vi "Calib_read_files.vi"   [LabVIEW 2013]
uses:
  Globals/Calib_global.vi
types:
  T1 = typedef "Cal_Inst_type.ctl" = enum16{"Propeller anemometer", "Pressure Transducer", "Hot wire", "Cross wire velocity", "Cross wire angle", "Generic Linear", "Generic Polynomial", "Generic BackPoly", "Fast FID", "Thermocouple", "Cold wire", "Pulsed Wire"}
  T2 = typedef "TypeCalib.ctl" = cluster{"high limit (10V)":sgl, "low limit (-10V)":sgl, "Ch No":i16, "Var name":string, "DAQmx Chan":tag}
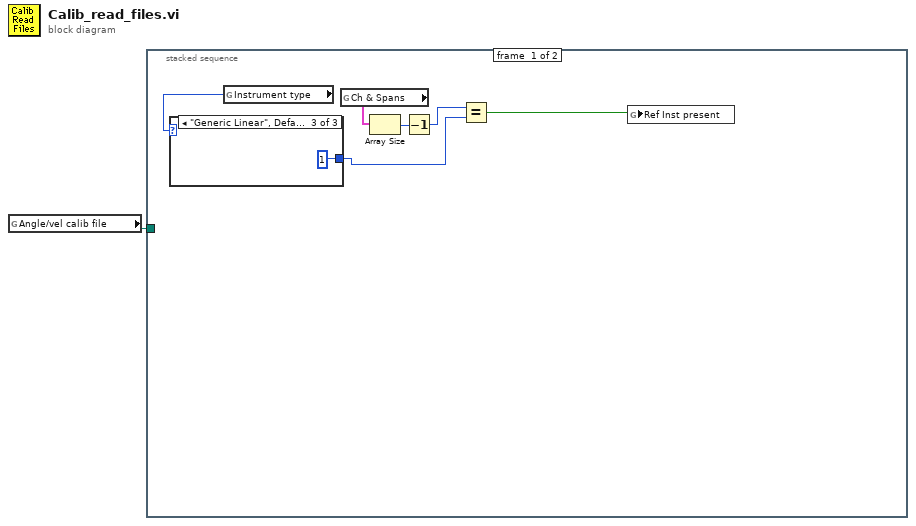
[diagram p0: block diagram]
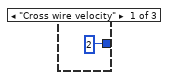
[diagram p2: hidden frame]
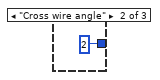
[diagram p3: hidden frame]
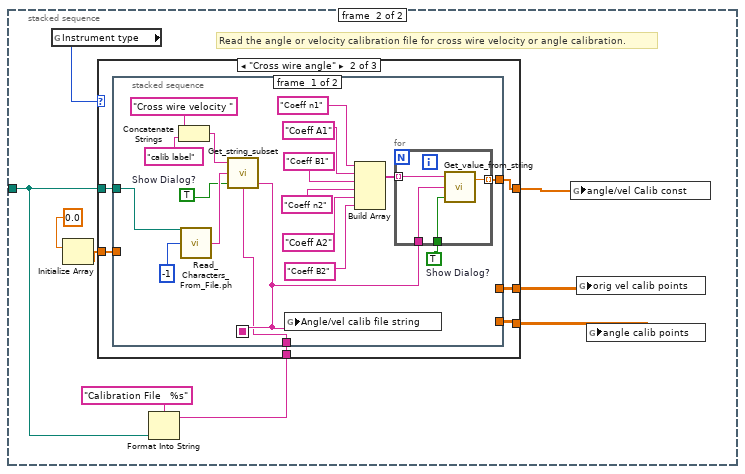
[diagram p4: hidden frame]
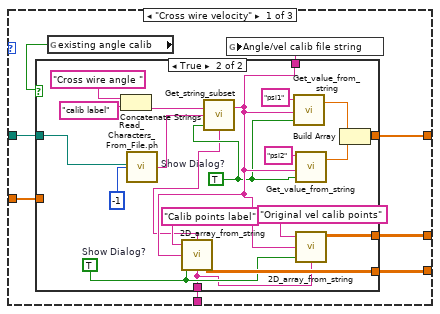
[diagram p5: hidden frame]
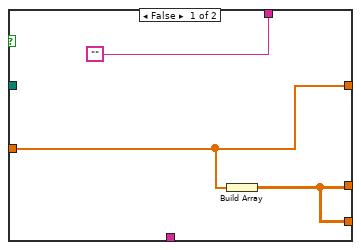
[diagram p6: hidden frame]
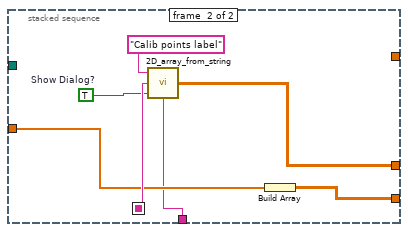
[diagram p7: hidden frame]
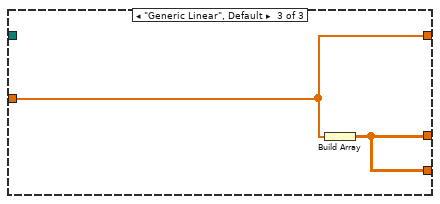
[diagram p8: hidden frame]
diagram:
  n1 = global read "Calib_global.vi" "Angle/vel calib file"() -> (w1:path)
  n2 = stacked-sequence {
    tunnel: w1 -> [_ w12]
    frame #0 {
      n3 = global read "Calib_global.vi" "Instrument type"() -> (w7:T1)
      n4 = case shown="\"Generic Linear\", Default" w7 {
        tunnel: [2 2 1] -> w2
        frame "Cross wire velocity" {
        }
        frame "Cross wire angle" {
        }
        frame "Generic Linear", Default {
        }
      }
      n5 = global read "Calib_global.vi" "Ch & Spans"() -> (w5:T2[])
      n6 = Array Size(array=w5) -> (size(s)=w6:i32)
      n7 = Decrement(x=w6) -> (x-1=w4:i32)
      n8 = Equal?(x=w4, y=w2) -> (x = y?=w3:bool)
      n9 = global write "Calib_global.vi" "Ref Inst present"(w3) -> ()
    }
    frame #1 {
      # "Read the angle or velocity calibration file for cross wire velocity or angle calibration."
      n10 = global read "Calib_global.vi" "Instrument type"() -> (w17:T1)
      n11 = Initialize Array(0.0) -> (w19:dbl[])  [unwired: 1 out]
      n12 = Format Into String(format string="Calibration File   %s", w12) -> (resulting string=w11:string)  [unwired: 2 in, 1 out]
      n13 = case shown="\"Cross wire angle\"" w17 {
        tunnel: [w27 w51 w86] -> w18
        tunnel: w19 -> [w26 w54 w86]
        tunnel: [w24 w55 w85] -> w14
        tunnel: [w25 w53 w85] -> w15
        tunnel: w12 -> [w21 w52 _]
        tunnel: w11 -> [w20 w50 _]
        frame "Cross wire velocity" {
          n14 = global read "Calib_global.vi" "existing angle calib"() -> (w23:bool)
          n15 = case shown="True" w23 {
            tunnel: [w30 w40] -> w27
            tunnel: w26 -> [w30 _]
            tunnel: [w29 w38] -> w25
            tunnel: [w29 w36] -> w24
            tunnel: ["" w35] -> w22
            tunnel: w21 -> [_ w34]
            tunnel: w20 -> [_ w31]
            frame False {
              n16 = Build Array(w30) -> (w29:dbl[][])
            }
            frame True {
              w32 = TRUE  # Show Dialog?
              w33 = TRUE  # Show Dialog?
              n17 = Concatenate Strings("Cross wire angle ", "calib label") -> (w41:string)
              n18 = call "Read_Characters_From_File.ph.vi"("file path (dialog if empty)"=w34, "number of characters (all:-1)"=-1) -> ("character string"=w43:string)  [unwired: 7 out]
              n19 = call "Get_string_subset.vi"("String Name"=w31, "Show Dialog?"=w33, "String to split"=w43, "File Label"=w41) -> ("Output string"=w35:string)  [unwired: 1 out]
              n20 = call "2D_array_from_string.vi"("String Name"=w31, "Show Dialog?"=w32, "Input string"=w35, "Array title"="Calib points label") -> ("2D data array"=w38:dbl[][])
              n21 = call "Get_value_from_string.vi"("Show Dialog?"=w33, "Input string"=w35, "Variable name"="psi1") -> ("Value"=w45:dbl)  [unwired: 1 out]
              n22 = call "Get_value_from_string.vi"("Show Dialog?"=w33, "Input string"=w35, "Variable name"="psi2") -> ("Value"=w44:dbl)  [unwired: 1 out]
              n23 = call "2D_array_from_string.vi"("String Name"=w31, "Show Dialog?"=w32, "Input string"=w35, "Array title"="Original vel calib points") -> ("2D data array"=w36:dbl[][])
              n24 = Build Array(w45, w44) -> (w40:dbl[])
            }
          }
          n25 = global write "Calib_global.vi" "Angle/vel calib file string"(w22) -> ()
        }
        frame "Cross wire angle" {
          n26 = stacked-sequence {
            seq-local: [w59 _] -> [_ w83]
            tunnel: [_ w82] -> w55
            tunnel: w54 -> [_ w81]
            tunnel: [_ w80] -> w53
            tunnel: w52 -> [w68 _]
            tunnel: [w60 _] -> w51
            tunnel: w50 -> [w56 w78]
            frame #0 {
              w57 = TRUE  # Show Dialog?
              w58 = TRUE  # Show Dialog?
              n27 = Concatenate Strings("Cross wire velocity ", "calib label") -> (w69:string)
              n28 = call "Read_Characters_From_File.ph.vi"("file path (dialog if empty)"=w68, "number of characters (all:-1)"=-1) -> ("character string"=w71:string)  [unwired: 7 out]
              n29 = call "Get_string_subset.vi"("String Name"=w56, "Show Dialog?"=w57, "String to split"=w71, "File Label"=w69) -> ("Output string"=w59:string)  [unwired: 1 out]
              n30 = global write "Calib_global.vi" "Angle/vel calib file string"(w59) -> ()
              n31 = Build Array("Coeff n1", "Coeff A1", "Coeff B1", "Coeff n2", "Coeff A2", "Coeff B2") -> (w61:string[])
              n32 = for {
                tunnel: w61 -> [w77] mode=indexing
                tunnel: w59 -> [w76]
                tunnel: [w75] -> w60 mode=indexing
                tunnel: w58 -> [w74]
                n33 = call "Get_value_from_string.vi"("Show Dialog?"=w74, "Input string"=w76, "Variable name"=w77) -> ("Value"=w75:dbl)  [unwired: 1 out]
              }
            }
            frame #1 {
              w79 = TRUE  # Show Dialog?
              n34 = call "2D_array_from_string.vi"("String Name"=w78, "Show Dialog?"=w79, "Input string"=w83, "Array title"="Calib points label") -> ("2D data array"=w82:dbl[][])
              n35 = Build Array(w81) -> (w80:dbl[][])
            }
          }
        }
        frame "Generic Linear", Default {
          n36 = Build Array(w86) -> (w85:dbl[][])
        }
      }
      n37 = global write "Calib_global.vi" "angle/vel Calib const"(w18) -> ()
      n38 = global write "Calib_global.vi" "orig vel calib points"(w14) -> ()
      n39 = global write "Calib_global.vi" "angle calib points"(w15) -> ()
    }
  }
